vi "Keithley 27XX Performance.vi"() -> ()   [LabVIEW 2020]
doc: "This VI shows a few ways to optimize the performance when taking large amounts of measurements."
uses:
  <instrlib>/Keithley 27XX/Public/Data/Read Multiple Direct.vi
  <instrlib>/Keithley 27XX/Keithley 27XX.lvlib
panel:
  in  "Serial Configuration":T1={"Baud Rate (9600)"=9600, "Flow Control (1: XON/XOFF)"=1, "Termination Char (0:CR)"=0} {"Termination Char (0:CR)" items=["CR", "LF"]; "Flow Control (1: XON/XOFF)" items=["None", "XON/XOFF", "RTS/CTS (2701 Only)", "XON/XOFF & RTS/CTS (2701 Only)"]; "Baud Rate (9600)" items=["300"=300, "600"=600, "1200"=1200, "2400"=2400, "4800"=4800, "9600"=9600, "19.2k"=19200, "38.4k (2701 Only)"=38400, "57.6k (2701 Only)"=57600, "115.2k (2701 Only)"=115200]}
  in  "Timeout (30000 milliseconds)":u32=30000
  in  "Sample Count (100)":i32=100
  out "Measurement Data":dbl[](array[numeric])
  in  "Function (0: DC Voltage)":u16(ring) items=["DC Voltage", "AC Voltage", "DC Current", "AC Current", "Resistance", "Four-Wire Resistance", "Temperature (C)", "Frequency", "Period", "Continuity"]
  in  "Channel List (101:110)":string="101:110"
  in  "VISA resource name":refnum<visa-resource-name>
  # "© 2005 National Instruments Corporation.  ALL RIGHTS RESERVED."
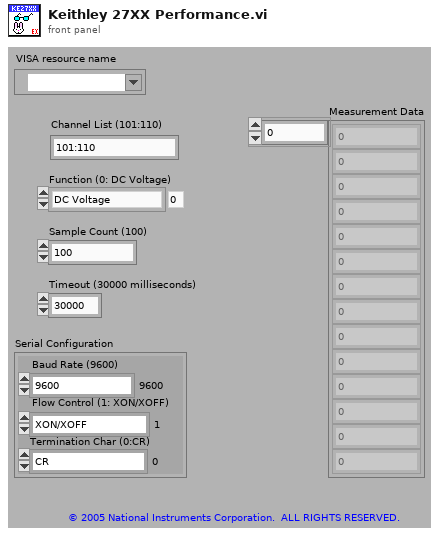
[diagram p1: front panel]
types:
  T1 = cluster{"Baud Rate (9600)":u32, "Flow Control (1: XON/XOFF)":u16, "Termination Char (0:CR)":u16}
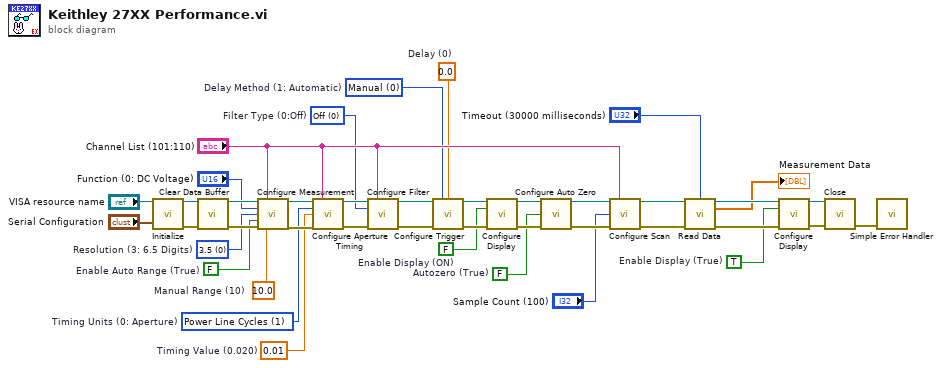
[diagram p0: block diagram]
diagram:
  w3 = 0.0  # Delay (0)
  w4 = TRUE  # Enable Display (True)
  w13 = 10.0  # Manual Range (10)
  w15 = u16 0 items=["Manual", "Automatic"]  # Delay Method (1: Automatic)
  w14 = u16 0 items=["Off", "Moving", "Repeat"]  # Filter Type (0:Off)
  w22 = u16 1 items=["Aperture", "Power Line Cycles"]  # Timing Units (0: Aperture)
  w25 = FALSE  # Enable Auto Range (True)
  w26 = u16 0 items=["3.5", "4.5", "5.5", "6.5"]  # Resolution (3: 6.5 Digits)
  w27 = 0.01  # Timing Value (0.020)
  w32 = FALSE  # Autozero (True)
  w35 = FALSE  # Enable Display (ON)
  n1 = call <instrlib>:"Initialize.vi"("VISA resource name"="VISA resource name", "Serial Configuration"="Serial Configuration") -> ("VISA resource name out"=w24:refnum<visa-resource-name>, "error out"=w23:errorcluster)  [unwired: 12 in]
  n2 = call <instrlib>:"Clear Data Buffer.vi"("VISA resource name"=w24, "error in (no error)"=w23) -> ("VISA resource name out"=w40:refnum<visa-resource-name>, "error out"=w39:errorcluster)  [unwired: 12 in]
  n3 = call <instrlib>:"Configure Measurement.vi"("VISA resource name"=w40, "Scan List (Empty)"="Channel List (101:110)", "Function (0: DC Voltage)"="Function (0: DC Voltage)", "Resolution (3: 6.5 Digits)"=w26, "Enable Auto Range (True)"=w25, "error in (no error)"=w39, "Manual Range (10)"=w13) -> ("VISA resource name out"=w29:refnum<visa-resource-name>, "error out"=w28:errorcluster)  [unwired: 7 in]
  n4 = call <instrlib>:"Configure Aperture Timing.vi"("VISA resource name"=w29, "Scan List (Empty)"="Channel List (101:110)", "Timing Units (0: Seconds)"=w22, "Timing Value (0.020)"=w27, "error in (no error)"=w28) -> ("VISA resource name out"=w21:refnum<visa-resource-name>, "error out"=w20:errorcluster)  [unwired: 9 in]
  n5 = call <instrlib>:"Configure Filter.vi"("VISA resource name"=w21, "Scan List (Empty)"="Channel List (101:110)", "Filter Type (0:Off)"=w14, "error in (no error)"=w20) -> ("VISA resource name out"=w18:refnum<visa-resource-name>, "error out"=w17:errorcluster)  [unwired: 10 in]
  n6 = call <instrlib>:"Configure Trigger.vi"("VISA resource name"=w18, "Delay Method (1: Automatic)"=w15, "Delay (0)"=w3, "error in (no error)"=w17) -> ("VISA resource name out"=w19:refnum<visa-resource-name>, "error out"=w41:errorcluster)  [unwired: 10 in]
  n7 = call <instrlib>:"Configure Display.vi"("VISA resource name"=w19, "Enable Display (True)"=w35, "error in (no error)"=w41) -> ("VISA resource name out"=w33:refnum<visa-resource-name>, "error out"=w34:errorcluster)  [unwired: 11 in]
  n8 = call <instrlib>:"Configure Auto Zero.vi"("VISA resource name"=w33, "Enable Auto Zero (True)"=w32, "error in (no error)"=w34) -> ("VISA resource name out"=w8:refnum<visa-resource-name>, "error out"=w7:errorcluster)  [unwired: 11 in]
  n9 = call <instrlib>:"Configure Scan.vi"("VISA resource name"=w8, "Channel List (101:110)"="Channel List (101:110)", "Sample Count (100)"="Sample Count (100)", "error in (no error)"=w7) -> ("VISA resource name out"=w12:refnum<visa-resource-name>, "error out"=w11:errorcluster)  [unwired: 10 in]
  n10 = call-poly <instrlib>:"Read Data.vi"("VISA resource name"=w12, "Timeout (30000 milliseconds)"="Timeout (30000 milliseconds)", "error in (no error)"=w11) -> ("VISA resource name out"=w9:refnum<visa-resource-name>, "Measurement Data"=→"Measurement Data":dbl[], "error out"=w10:errorcluster)  [unwired: 7 in, 3 out]
  n11 = call <instrlib>:"Configure Display.vi"("VISA resource name"=w9, "Enable Display (True)"=w4, "error in (no error)"=w10) -> ("VISA resource name out"=w31:refnum<visa-resource-name>, "error out"=w30:errorcluster)  [unwired: 11 in]
  n12 = call <instrlib>:"Close.vi"("VISA resource name"=w31, "error in (no error)"=w30) -> ("error out"=w36:errorcluster)  [unwired: 13 in]
  n13 = call <vilib>:"Simple Error Handler.vi"("error in (no error)"=w36) -> ()  [unwired: 4 in, 5 out]
